vi "ROI entry-Dwell time switch.vi"(8 "error in (no error)":errorcluster, 11 "ROI Enum":T1) -> (0 "error out":errorcluster)   [LabVIEW 2020]
uses:
  Typedefs/ROI ID Enum.ctl
  Globals/gl_ROI Entry UI globals.vi
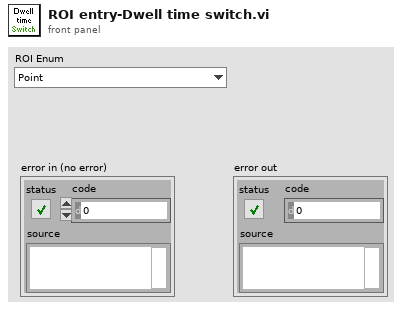
[diagram p1: front panel]
types:
  T1 = typedef "ROI ID Enum.ctl" = enum16{"Point", "MiniScan", "Comp. MiniScan", "Rectangle", "Comp. volume", "Arb. plane point", "None"}
  T2 = typedef "ROI entry screen ctrl refs cluster.ctl" = cluster{"Done button":refnum<vi>, "Imaging button":refnum<vi>, "Acquisition button":refnum<vi>, "Scan dwell time per pixel (us)":refnum<vi>, "# of planes":refnum<vi>, "Zoom Ctrl":refnum<vi>, "Equal size":refnum<vi>, "Channel":refnum<vi>, "Image Display":refnum<vi>, "Z-Plane Selector":refnum<vi>, "Number of lines left":refnum<vi>, "Z-stack folder path":refnum<vi>, "POI Density":refnum<vi>, "Arb Plane Entry":refnum<vi>, "Whole Plane":refnum<vi>, "Line Mode":refnum<vi>, "Clear Last":refnum<vi>, "Clear All":refnum<vi>, "Delete Lines":refnum<vi>, "Trial Length (sec)":refnum<vi>, "Palette Type":refnum<vi>, "Intensity slider":refnum<vi>, "# POI":refnum<vi>, "Max Z Proj":refnum<vi>, "Zplane ind":refnum<vi>, "Wavelength (nm)":refnum<vi>, "Number of Trials":refnum<vi>, "Funct stim.trig.enable":refnum<vi>, "Funct stim.trig.delay (s)":refnum<vi>, "Line Mode":refnum<vi>, "Step size (µm)":refnum<vi>, "ROI move mode":refnum<vi>, "Cool-down time (s)":refnum<vi>, "Enable cool-down time":refnum<vi>, "Motor Z ind. (um)":refnum<vi>, "AOL Z ind. (um)":refnum<vi>, "Load Reference Image":refnum<vi>, "Rel.  Res.":refnum<vi>, "ROI LIST":refnum<vi>, "Show All":refnum<vi>, "ROI Type":refnum<vi>, "Start Plane":refnum<vi>, "Stop Plane":refnum<vi>, "Offset ROI":refnum<vi>, "Tab Control":refnum<vi>, "Laser Power(%)":refnum<vi>, "Cycle rate":refnum<vi>, "FOV (Ind.)":refnum<vi>, "Frame Size (Ind.)":refnum<vi>, "Resolution (Ind.)":refnum<vi>, "Pixel Density (Ind)":refnum<vi>, "Laser Power (Ind.)":refnum<vi>, "Dwell Time (Ind.)":refnum<vi>, "Adj MC":refnum<vi>}
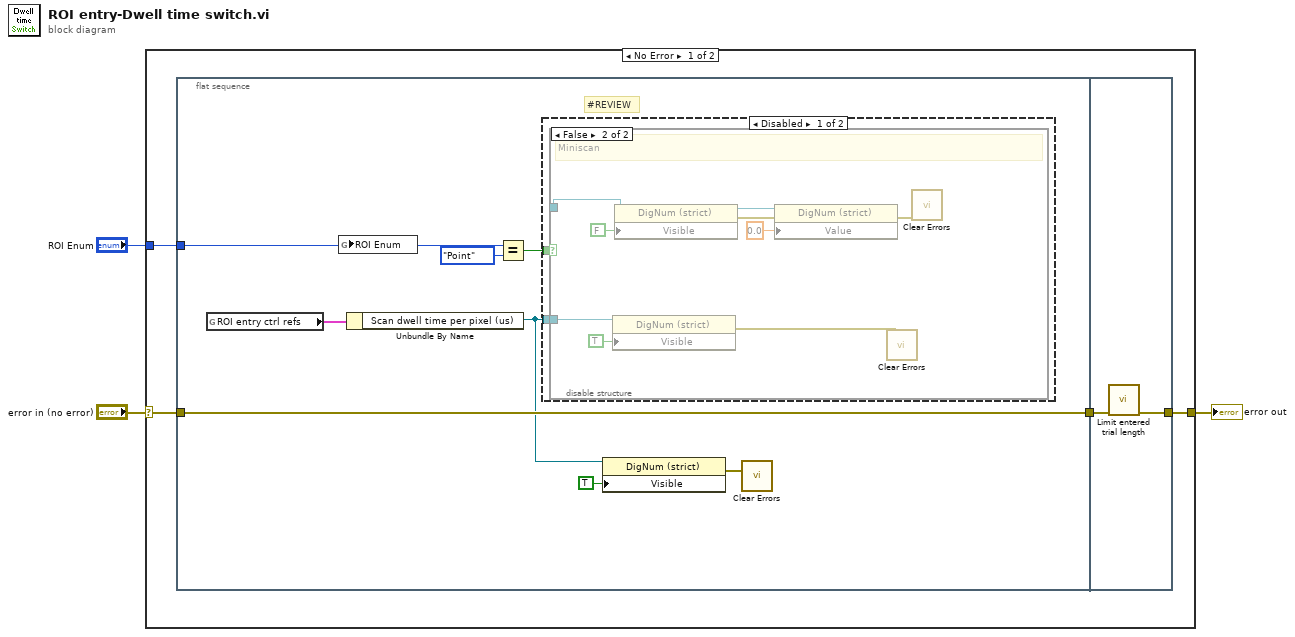
[diagram p0: block diagram]
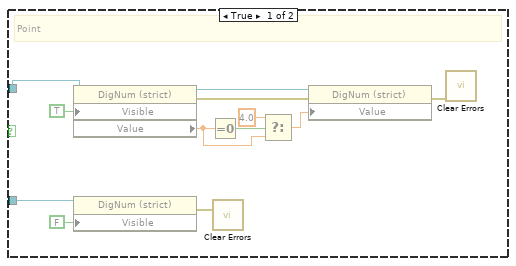
[diagram p2: hidden frame]
diagram:
  n1 = case shown="No Error" "error in (no error)" {
    selector: "error in (no error)" -> [w5 w41]
    tunnel: "ROI Enum" -> [w7 _]
    tunnel: [w4 w41] -> w1
    frame No Error {
      n2 = flat-sequence {
        tunnel: w7 -> [w12]
        tunnel: [w11] -> w6
        tunnel: w5 -> [w11]
        tunnel: w6 -> [w40]
        tunnel: [w39] -> w4
        frame #0 {
          # "#REVIEW"
          n3 = global read "gl_ROI Entry UI globals.vi" "ROI entry ctrl refs"() -> (w14:T2)
          n4 = global write "gl_ROI Entry UI globals.vi" "ROI Enum"(w12) -> ()
          n5 = Unbundle By Name(w14) -> ("Scan dwell time per pixel (us)"=w8:refnum<vi>)
          n6 = Equal?(x=w12, y=ROI_ID_Enum."Point") -> (x = y?=w13:bool)
          n7 = disable-structure shown="Disabled" {
            disable-tunnel: w8 -> [w17 _]
            disable-tunnel: w13 -> [w16 _]
            frame Disabled {
              n8 = case shown="False" w16 {
                tunnel: w17 -> [w29 w38]
                tunnel: _ -> [w28 w37]
                frame True {
                  # "Point"
                  n9 = property on="Property Node" class="DigNum (strict)"(reference=w28, "Visible"=TRUE) -> (reference out=w23:refnum<vi>, error out=w24:errorcluster, "Value"=w18:dbl)  [unwired: 1 in]
                  n10 = property on="Property Node" class="DigNum (strict)"(reference=w29, "Visible"=FALSE) -> (error out=w27:errorcluster)  [unwired: 1 in, 1 out]
                  n11 = Equal To 0?(x=w18) -> (x = 0?=w21:bool)
                  n12 = call <vilib>:"Clear Errors.vi"("error in (no error)"=w27) -> ()  [unwired: 5 in, 2 out]
                  n13 = Select(t=4.0, s=w21, f=w18) -> (s? t:f=w19:dbl)
                  n14 = property on="Property Node" class="DigNum (strict)"(reference=w23, error in=w24, "Value"=w19) -> (error out=w22:errorcluster)  [unwired: 1 out]
                  n15 = call <vilib>:"Clear Errors.vi"("error in (no error)"=w22) -> ()  [unwired: 5 in, 2 out]
                }
                frame False {
                  # "Miniscan"
                  n16 = property on="Property Node" class="DigNum (strict)"(reference=w38, "Visible"=TRUE) -> (error out=w36:errorcluster)  [unwired: 1 in, 1 out]
                  n17 = property on="Property Node" class="DigNum (strict)"(reference=w37, "Visible"=FALSE) -> (reference out=w32:refnum<vi>, error out=w33:errorcluster)  [unwired: 1 in]
                  n18 = property on="Property Node" class="DigNum (strict)"(reference=w32, error in=w33, "Value"=0.0) -> (error out=w31:errorcluster)  [unwired: 1 out]
                  n19 = call <vilib>:"Clear Errors.vi"("error in (no error)"=w36) -> ()  [unwired: 5 in, 2 out]
                  n20 = call <vilib>:"Clear Errors.vi"("error in (no error)"=w31) -> ()  [unwired: 5 in, 2 out]
                }
              }
            }
            frame Enabled {
            }
          }
          n21 = property on="Property Node" class="DigNum (strict)"(reference=w8, "Visible"=TRUE) -> (error out=w10:errorcluster)  [unwired: 1 in, 1 out]
          n22 = call <vilib>:"Clear Errors.vi"("error in (no error)"=w10) -> ()  [unwired: 5 in, 2 out]
        }
        frame #1 {
          n23 = call "Limit entered trial length.vi"("error in (no error)"=w40) -> ("error out"=w39:errorcluster)  [unwired: 10 in]
        }
      }
    }
    frame Error {
    }
  }
  "error out" <- w1
